vi "Plot Bezier Curve.vi"() -> ()   [LabVIEW 2019]
panel:
  out "x-y 3":u32
  out "l":dbl
  out "l total":dbl
  out "Array 3":sgl[](array[numeric])
  out "Array 2":sgl[](array[numeric])
  out "Array":dbl[](array[numeric])
  out "Curve Graph 5":cluster{"X":dbl[], "Y":dbl[]}(graph)
  out "x-y 2":u32
  out "Curve Graph 3":cluster{sgl, sgl}[](graph)
  out "Curve Graph 2":cluster{sgl, sgl}[](graph)
  out "Curvature":dbl[](graph)
  out "appended array":cluster{"x":dbl, "y":dbl}[](array[cluster])
  out "d2 ctrl pts":cluster{dbl, dbl}[](array[cluster])
  out "2nd derivative":cluster{"x":sgl, "y":sgl}[](graph)
  out "1st derivative":cluster{"x":sgl, "y":sgl}[](graph)
  out "d ctrl pts":cluster{dbl, dbl}[](array[cluster])
  out "size(s)":i32
  out "Curve Graph":cluster{"x":sgl, "y":sgl}[](graph)
  out "x-y":u32
  in  "percision":dbl=0.01
  in  "ctrl points":cluster{dbl, dbl}[](array[cluster])
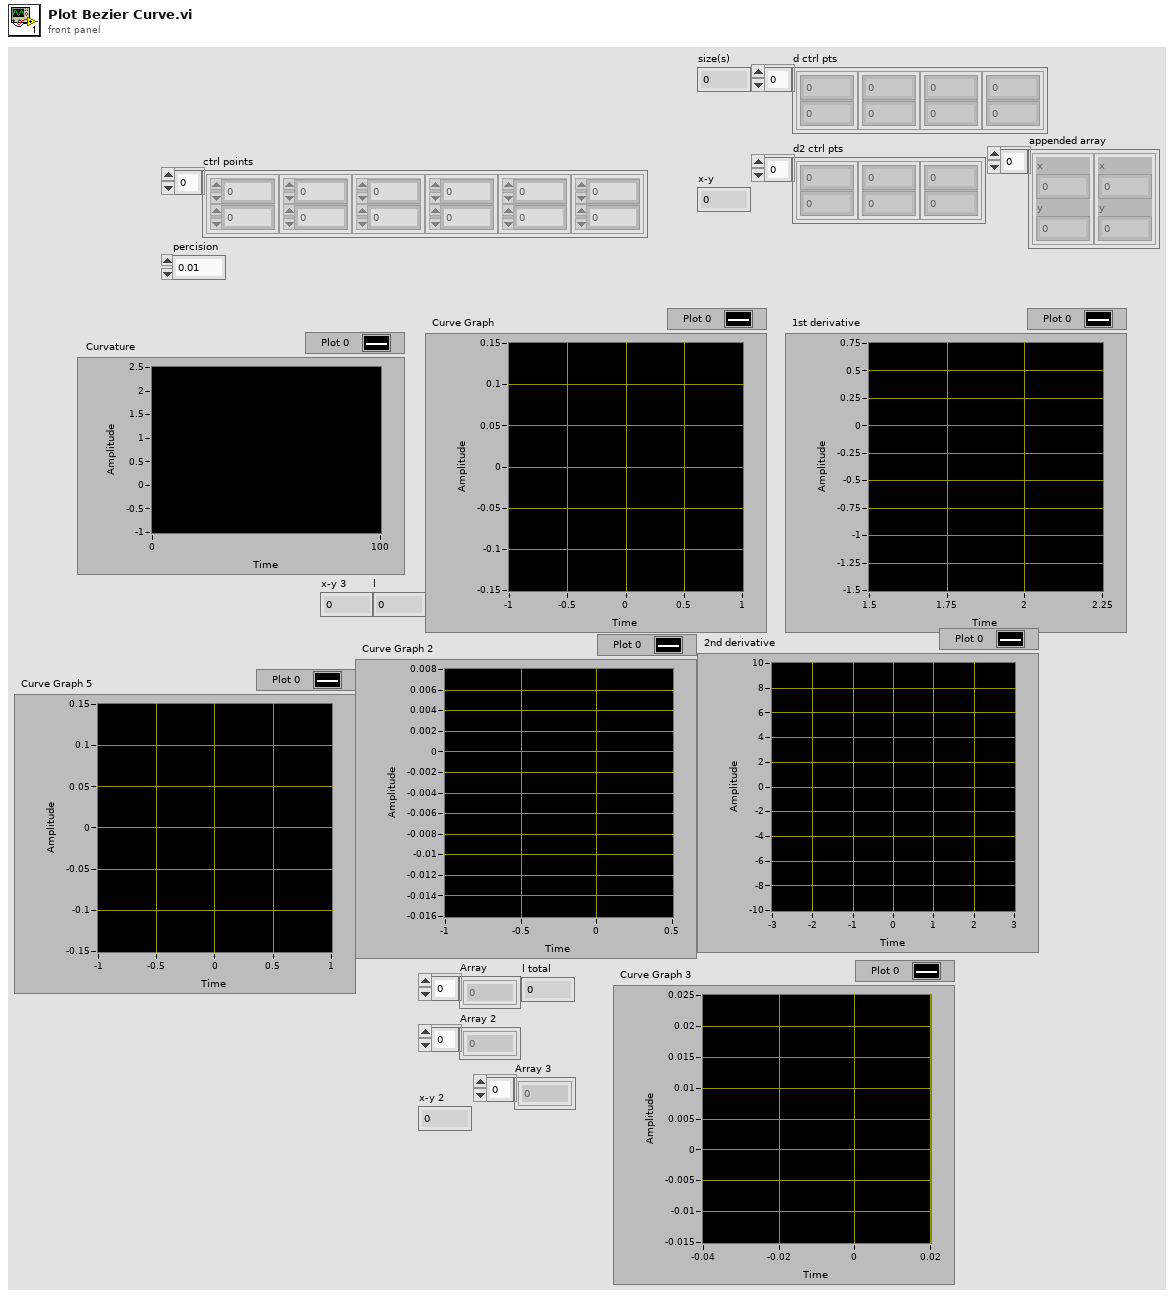
[diagram p1: front panel]
types:
  T1 = typedef "Bezier Curve.ctl" = cluster{"x":sgl, "y":sgl}[]
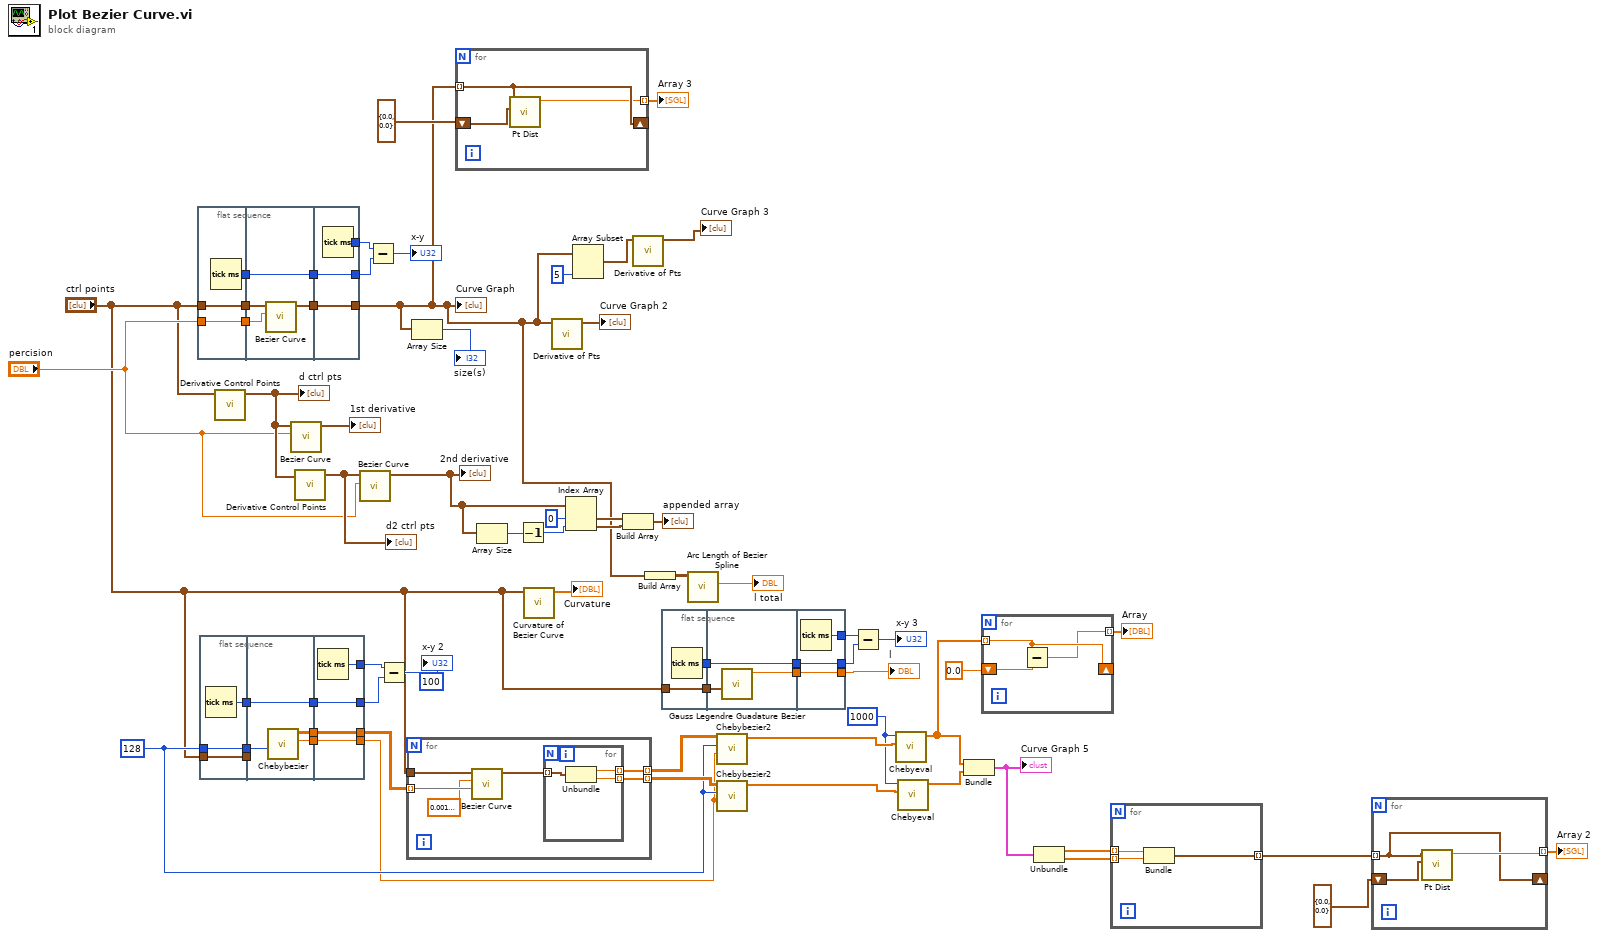
[diagram p0: block diagram]
diagram:
  w25 = u32 1000 ("number of points")
  (unwired) u32 100 ("number of points")
  w30 = u32 128 ("order")
  n1 = flat-sequence {
    tunnel: "percision" -> [w68]
    tunnel: "ctrl points" -> [w69]
    tunnel: [w69] -> w65
    tunnel: [w68] -> w64
    tunnel: [w67] -> w60
    tunnel: [w70] -> w66
    tunnel: w65 -> [w73]
    tunnel: w64 -> [w71]
    tunnel: [w72] -> w61
    tunnel: w60 -> [w72]
    tunnel: [w76] -> w11
    tunnel: w66 -> [w76]
    tunnel: [w75] -> w63
    tunnel: [w74] -> w62
    tunnel: w61 -> [w74]
    frame #0 {
      n2 = Tick Count (ms)() -> (millisecond timer value=w67:u32)
    }
    frame #1 {
      n3 = call "Bezier Curve.vi"("percision"=w71, "ctrl points"=w73) -> ("curve"=w70:T1)  [unwired: 9 in]
    }
    frame #2 {
      n4 = Tick Count (ms)() -> (millisecond timer value=w75:u32)
    }
  }
  n5 = flat-sequence {
    tunnel: w30 -> [w78]
    tunnel: "ctrl points" -> [w79]
    tunnel: [w79] -> w41
    tunnel: [w78] -> w40
    tunnel: [w77] -> w36
    tunnel: w41 -> [_]
    tunnel: w40 -> [w83]
    tunnel: [w82] -> w37
    tunnel: w36 -> [w82]
    tunnel: [w81] -> w33
    tunnel: [w80] -> w29
    tunnel: [w87] -> w39
    tunnel: [w86] -> w38
    tunnel: w37 -> [w86]
    tunnel: [w85] -> w34
    tunnel: w33 -> [w85]
    tunnel: [w84] -> w28
    tunnel: w29 -> [w84]
    frame #0 {
      n6 = Tick Count (ms)() -> (millisecond timer value=w77:u32)
    }
    frame #1 {
      n7 = call "Chebybezier.vi"("order"=w83) -> ("x/y"=w80:dbl, "X values"=w81:dbl[][])  [unwired: 9 in]
    }
    frame #2 {
      n8 = Tick Count (ms)() -> (millisecond timer value=w87:u32)
    }
  }
  n9 = call "Derivative Control Points.vi"("ctrl points"="ctrl points") -> ("d ctrl pts"=w56:cluster{dbl, dbl}[])  [unwired: 10 in]
  "d ctrl pts" <- w56
  n10 = call "Bezier Curve.vi"("percision"="percision", "ctrl points"=w56) -> ("curve"=→"1st derivative":T1)  [unwired: 9 in]
  n11 = call "Derivative Control Points.vi"("ctrl points"=w56) -> ("d ctrl pts"=w55:cluster{dbl, dbl}[])  [unwired: 10 in]
  "d2 ctrl pts" <- w55
  n12 = call "Bezier Curve.vi"("percision"="percision", "ctrl points"=w55) -> ("curve"=w54:T1)  [unwired: 9 in]
  "2nd derivative" <- w54
  n13 = Subtract(x=w63, y=w62) -> (x-y=→"x-y":u32)
  n14 = Subtract(x=w39, y=w38) -> (x-y=→"x-y 2":u32)
  n15 = for {
    tunnel: w34 -> [w93] mode=indexing
    tunnel: "ctrl points" -> [w92]
    tunnel: [w89] -> w31 mode=indexing
    tunnel: [w88] -> w32 mode=indexing
    n16 = call "Bezier Curve.vi"("position"=w93, "percision"=sgl 0.001, "ctrl points"=w92) -> ("curve"=w90:T1)  [unwired: 8 in]
    n17 = for {
      tunnel: w90 -> [w96] mode=indexing
      tunnel: [w95] -> w88 mode=indexing
      tunnel: [w94] -> w89 mode=indexing
      n18 = Unbundle(w96) -> ("x"=w94:sgl, "y"=w95:sgl)
    }
  }
  n19 = Array Size(array=w11) -> (size(s)=→"size(s)":i32)
  n20 = for {
    tunnel: w11 -> [w98] mode=indexing
    shift-right: [w98] -> _
    shift-left: cluster{"x":sgl, "y":sgl} {"x"=0.0, "y"=0.0} ("element") -> [w99]
    tunnel: [w97] -> w13 mode=indexing
    n21 = call "Pt Dist.vi"("point b"=w99, "point a"=w98) -> ("dist"=w97:sgl)  [unwired: 9 in]
  }
  "Array 3" <- w13
  n22 = Array Size(array=w54) -> (size(s)=w53:i32)
  n23 = Decrement(x=w53) -> (x-1=w52:i32)
  n24 = call "Curvature of Bezier Curve.vi"("curve"="ctrl points") -> ("curvature"=→"Curvature":dbl[])  [unwired: 10 in]
  n25 = call "Derivative of Pts.vi"("pts"=w11) -> ("pts out"=→"Curve Graph 2":cluster{sgl, sgl}[])  [unwired: 10 in]
  n26 = Index Array(array=w54, index #1=0 ("index"), index #2=w52) -> (element #1=w50:cluster{"x":sgl, "y":sgl}, element #2=w49:cluster{"x":sgl, "y":sgl})
  n27 = Array Subset(array=w11, length=5) -> (w43:T1)  [unwired: 1 in]
  n28 = Build Array(w50, w49) -> (→"appended array":cluster{"x":sgl, "y":sgl}[])
  n29 = call "Derivative of Pts.vi"("pts"=w43) -> ("pts out"=→"Curve Graph 3":cluster{sgl, sgl}[])  [unwired: 10 in]
  n30 = Build Array(w11) -> (w10:cluster{"x":sgl, "y":sgl}[][])
  n31 = flat-sequence {
    tunnel: "ctrl points" -> [w101]
    tunnel: [w101] -> w6
    tunnel: [w100] -> w2
    tunnel: [w103] -> w7
    tunnel: w6 -> [w104]
    tunnel: [w102] -> w3
    tunnel: w2 -> [w102]
    tunnel: [w107] -> w8
    tunnel: w7 -> [w107]
    tunnel: [w106] -> w5
    tunnel: [w105] -> w4
    tunnel: w3 -> [w105]
    frame #0 {
      n32 = Tick Count (ms)() -> (millisecond timer value=w100:u32)
    }
    frame #1 {
      n33 = call "Gauss Legendre Guadature Bezier.vi"("ctrl points"=w104) -> ("l"=w103:dbl)  [unwired: 10 in]
    }
    frame #2 {
      n34 = Tick Count (ms)() -> (millisecond timer value=w106:u32)
    }
  }
  n35 = call "Arc Length of Bezier Spline.vi"("bezier spline"=w10) -> ("l total"=→"l total":dbl)  [unwired: 8 in, 2 out]
  n36 = call "Chebybezier2.vi"("Numeric"=w28, "order"=w30, "Y"=w31) -> ("C"=w26:dbl[])  [unwired: 8 in]
  n37 = call "Chebybezier2.vi"("Numeric"=w28, "order"=w30, "Y"=w32) -> ("C"=w27:dbl[])  [unwired: 8 in]
  n38 = Subtract(x=w5, y=w4) -> (x-y=→"x-y 3":u32)
  n39 = call "Chebyeval.vi"("C"=w26, "number of points"=w25) -> ("Y"=w23:dbl[])  [unwired: 8 in, 1 out]
  n40 = call "Chebyeval.vi"("C"=w27, "number of points"=w25) -> ("Y"=w24:dbl[])  [unwired: 8 in, 1 out]
  n41 = Bundle("Y"=w23, "Y"=w24) -> (w20:cluster{"Y":dbl[], "Y":dbl[]})  [unwired: 1 in]
  "Curve Graph 5" <- w20
  n42 = for {
    tunnel: w23 -> [w109] mode=indexing
    shift-right: [w109] -> _
    shift-left: 0.0 -> [w110]
    tunnel: [w108] -> w21 mode=indexing
    n43 = Subtract(x=w109, y=w110) -> (x-y=w108:dbl)
  }
  "Array" <- w21
  n44 = Unbundle(w20) -> ("Y"=w19:dbl[], "Y"=w18:dbl[])
  n45 = for {
    tunnel: w19 -> [w113] mode=indexing
    tunnel: w18 -> [w112] mode=indexing
    tunnel: [w111] -> w17 mode=indexing
    n46 = Bundle(w113, w112) -> (w111:cluster{dbl, dbl})  [unwired: 1 in]
  }
  n47 = for {
    tunnel: w17 -> [w114] mode=indexing
    shift-right: [w114] -> _
    shift-left: cluster{dbl, dbl} {0.0, 0.0} ("element") -> [w116]
    tunnel: [w115] -> w15 mode=indexing
    n48 = call "Pt Dist.vi"("point b"=w116, "point a"=w114) -> ("dist"=w115:sgl)  [unwired: 9 in]
  }
  "Array 2" <- w15
  "Curve Graph" <- w11
  "l" <- w8
